vi "Command_Rotate.vi"(7 "Parameters":dbl[](array[numeric]), 11 "Startup":bool) -> (4 "Completed":bool, 6 "Target_Drive_Powers":dbl[](array[numeric]), 10 "Target_Wheel_Angles":dbl[](array[numeric]), 15 "Reinit":bool)   [LabVIEW 2020]
uses:
  Auto Utilities/Command_Execution_State.ctl
  Globals/Sensor_Values.vi
panel:
  out "Initial_Y_Position(in)":dbl
  out "Initial_X_Position(in)":dbl
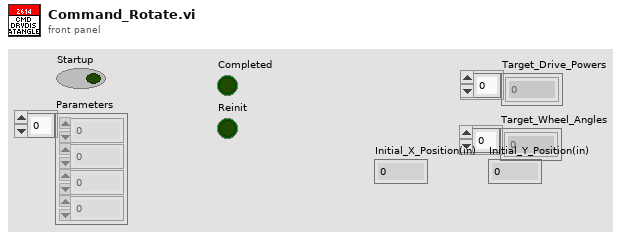
[diagram p1: front panel]
types:
  T1 = typedef "Command_Execution_State.ctl" = enum16{"Initialize", "Execute", "Finish"}
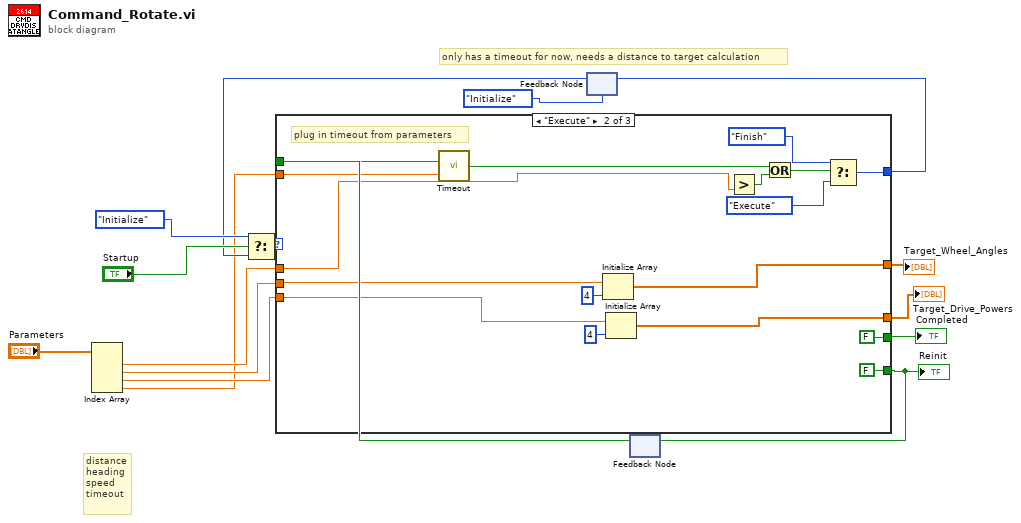
[diagram p0: block diagram]
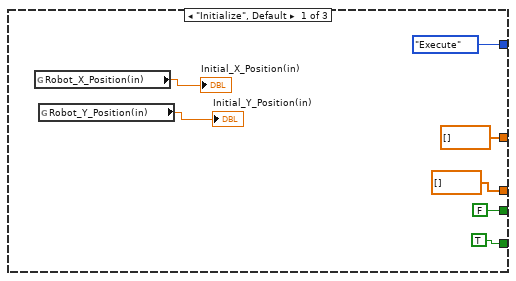
[diagram p2: hidden frame]
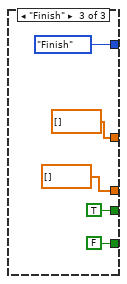
[diagram p3: hidden frame]
diagram:
  # "only has a timeout for now, needs a distance to target calculation"
  # "distance\nheading\nspeed\ntimeout"
  n1 = Index Array(array="Parameters") -> (element #1=w6:dbl, element #2=w5:dbl, element #3=w4:dbl, element #4=w3:dbl)  [unwired: 4 in]
  n2 = feedback #1(Command_Execution_State."Initialize") -> (w12:T1)
  n3 = Select(t=Command_Execution_State."Initialize", s="Startup", f=w12) -> (s? t:f=w14:T1)
  n4 = feedback #2() -> (w8:bool)  [unwired: 1 in]
  n5 = case shown="\"Execute\"" w14 {
    tunnel: [Command_Execution_State."Execute" w38 Command_Execution_State."Finish"] -> w13
    tunnel: [FALSE ("Reinit") FALSE ("Reinit") TRUE ("Reinit")] -> w10
    tunnel: [TRUE ("Reinit") FALSE ("Reinit") FALSE ("Reinit")] -> w9
    tunnel: w8 -> [_ w35 _]
    tunnel: w6 -> [_ w24 _]
    tunnel: w5 -> [_ w31 _]
    tunnel: w4 -> [_ w27 _]
    tunnel: w3 -> [_ w32 _]
    tunnel: [dbl[] [] w29 dbl[] []] -> w2
    tunnel: [dbl[] [] w26 dbl[] []] -> w1
    frame "Initialize", Default {
      n6 = global read "Sensor_Values.vi" "Robot_X_Position(in)"() -> (→"Initial_X_Position(in)":dbl)
      n7 = global read "Sensor_Values.vi" "Robot_Y_Position(in)"() -> (→"Initial_Y_Position(in)":dbl)
    }
    frame "Execute" {
      # "plug in timeout from parameters"
      n8 = call "Timeout.vi"("Timeout"=w32, "Initialize"=w35) -> ("Timed Out?"=w33:bool)
      n9 = Initialize Array(w31, 4 ("dimension size")) -> (w29:dbl[])
      n10 = Initialize Array(w27, 4 ("dimension size")) -> (w26:dbl[])
      n11 = Greater?(y=w24) -> (0:w25:bool)  [unwired: 1 in]
      n12 = Or(x=w33, y=w25) -> (x .or. y?=w34:bool)
      n13 = Select(t=Command_Execution_State."Finish", s=w34, f=Command_Execution_State."Execute") -> (s? t:f=w38:T1)
    }
    frame "Finish" {
    }
  }
  "Reinit" <- w9
  "Completed" <- w10
  "Target_Wheel_Angles" <- w2
  "Target_Drive_Powers" <- w1
  n14 = feedback-in #1(w13) -> ()
  n15 = feedback-in #2(w9) -> ()
